vi "Delete TargetPanel by NodeRef.vi"(8 "error in":errorcluster caption="错误输入（无错误）", 9 "Abort VI":bool=TRUE, 10 "Node*":refnum<data-value>, 11 "PanelRootNode 输入":refnum<class "PanelRootNode.lvclass"> caption="DNL_LabVIEW Object in") -> (0 "error out":errorcluster caption="错误输出", 3 "PanelRootNode 输出":refnum<class "PanelRootNode.lvclass"> caption="DNL_LabVIEW Object out")   [LabVIEW 2013, in "PanelRootNode.lvclass"]
uses:
  PanelRootNode.lvclass
  PanelObject/PanelObject.lvclass
  PanelLinkNode/PanelLinkNode.lvclass/PanelLinkNode.ctl
  PanelDataNode/PanelDataNode.lvclass
  PanelLinkNode/PanelLinkNode.lvclass
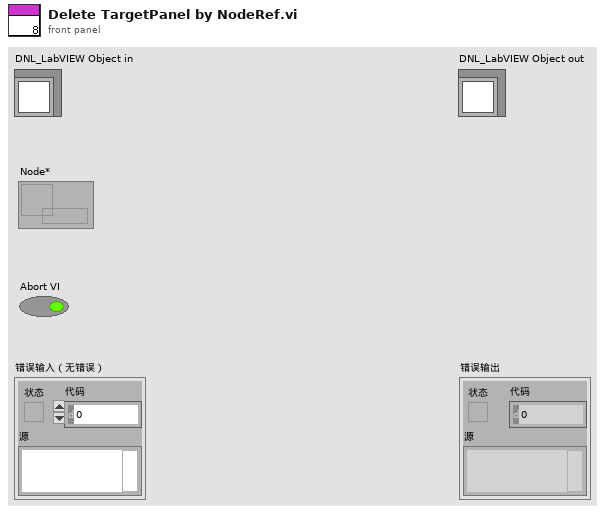
[diagram p1: front panel]
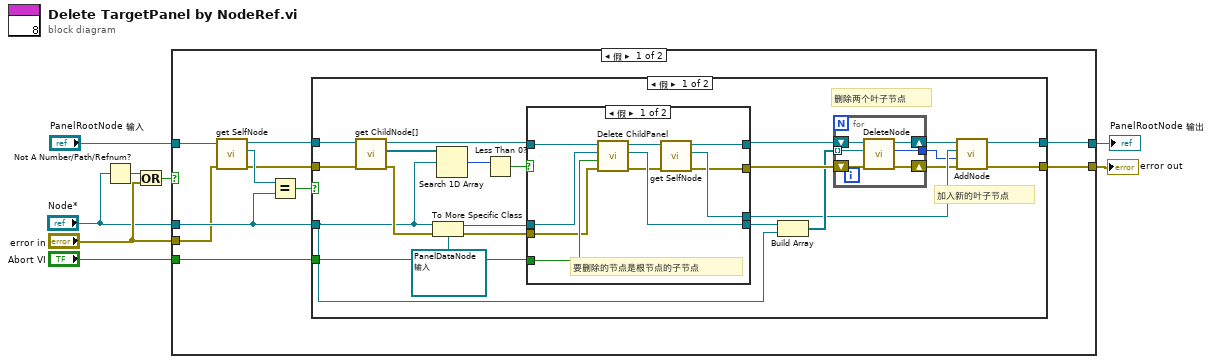
[diagram p0: block diagram]
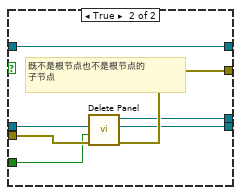
[diagram p2: hidden frame]
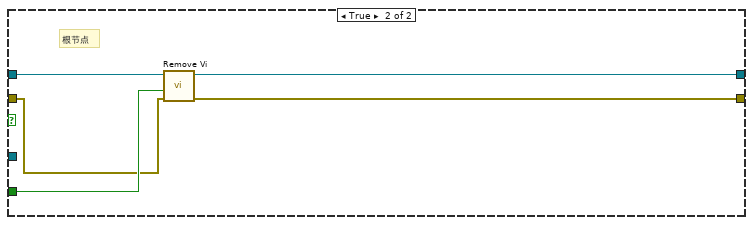
[diagram p3: hidden frame]
diagram:
  n1 = Not A Number/Path/Refnum?(number/path/refnum="Node*") -> (NaN/Path/Refnum?=w5:bool)
  n2 = Or(x=w5, y="error in") -> (x .or. y?=w4:bool)
  n3 = case shown="假" w4 {
    tunnel: [w10 w69] -> w8
    tunnel: [w14 w70] -> w6
    tunnel: "PanelRootNode 输入" -> [w18 w70]
    tunnel: "Node*" -> [w11 _]
    tunnel: "error in" -> [w9 w69]
    tunnel: "Abort VI" -> [w13 _]
    frame False {
      n4 = call "get SelfNode.vi"("error in (no error)"=w9, "PanelLinkNode输入"=w18) -> ("error out"=w12:errorcluster, "SelfNode*"=w17:refnum<data-value>, "PanelLinkNode输出"=w16:refnum<class "PanelRootNode.lvclass">)  [unwired: 7 in]
      n5 = Equal?(x=w17, y=w11) -> (x = y?=w15:bool)
      n6 = case shown="假" w15 {
        tunnel: w16 -> [w40 w68]
        tunnel: [w23 w67] -> w14
        tunnel: w13 -> [w34 w66]
        tunnel: w12 -> [w39 w64]
        tunnel: w11 -> [w27 _]
        tunnel: [w19 w65] -> w10
        frame False {
          # "加入新的叶子节点"
          # "删除两个叶子节点"
          n7 = call "get ChildNode[].vi"("error in (no error)"=w39, "PanelLinkNode输入"=w40) -> ("error out"=w31:errorcluster, "ChildNode*[]"=w38:refnum<data-value>[], "PanelLinkNode输出"=w36:refnum<class "PanelRootNode.lvclass">)  [unwired: 7 in]
          n8 = To More Specific Class(target class=refnum<data-value> refnum ("数据值引用"), reference=w27, error in=w31) -> (specific class reference=w32:refnum<data-value>, error out=w30:errorcluster)
          n9 = Search 1D Array(1D array=w38, element=w27) -> (index of element=w37:i32)  [unwired: 1 in]
          n10 = Less Than 0?(x=w37) -> (x < 0?=w35:bool)
          n11 = case shown="假" w35 {
            tunnel: w36 -> [w56 w63]
            tunnel: [w50 w63] -> w29
            tunnel: w32 -> [w55 w62]
            tunnel: w34 -> [w54 w59]
            tunnel: w30 -> [w53 w61]
            tunnel: [w47 w60] -> w26
            tunnel: [w52 w58] -> w28
            tunnel: [w49 w57] -> w22
            frame False {
              # "要删除的节点是根节点的子节点"
              n12 = call-dynamic "Delete ChildPanel.vi"("error in"=w53, "Abort VI"=w54, "ChildNode*"=w55, "ParentNode in"=w56) -> ("error out"=w48:errorcluster, "AnotherChildNode*"=w52:refnum<data-value>, "Parent out"=w51:refnum<class "PanelRootNode.lvclass">)  [unwired: 5 in]
              n13 = call "get SelfNode.vi"("error in (no error)"=w48, "PanelLinkNode输入"=w51) -> ("error out"=w47:errorcluster, "SelfNode*"=w49:refnum<data-value>, "PanelLinkNode输出"=w50:refnum<class "PanelRootNode.lvclass">)  [unwired: 7 in]
            }
            frame True {
              # "既不是根节点也不是根节点的\n子节点"
              n14 = call "Delete Panel.vi"("error in (no error)"=w61, "Abort VI"=w59, "SelfNode*"=w62) -> ("error out"=w60:errorcluster, "BrotherNodeBeDeleted"=w58:refnum<data-value>, "ParentNode*"=w57:refnum<data-value>)  [unwired: 6 in]
            }
          }
          n15 = Build Array(w28, w27) -> (w25:refnum<data-value>[])
          n16 = for {
            tunnel: w25 -> [w43] mode=indexing
            shift-right: [w45] -> w24
            shift-left: w29 -> [w46]
            shift-right: [w42] -> w20
            shift-left: w26 -> [w44]
            tunnel: [w41] -> w21
            n17 = call "DeleteNode.vi"("error in (no error)"=w44, "Node*"=w43, "PanelRootNode 输入"=w46) -> ("error out"=w42:errorcluster, "index"=w41:i32, "PanelRootNode 输出"=w45:refnum<class "PanelRootNode.lvclass">)  [unwired: 6 in]
          }
          n18 = call "AddNode.vi"("error in (no error)"=w20, "Index"=w21, "Node*"=w22, "PanelRootNode 输入"=w24) -> ("error out"=w19:errorcluster, "PanelRootNode 输出"=w23:refnum<class "PanelRootNode.lvclass">)  [unwired: 6 in]
        }
        frame True {
          # "根节点"
          n19 = call-dynamic "Remove Vi.vi"("error in"=w64, "Abort VI"=w66, "PanelDataNode 输入"=w68) -> ("error out"=w65:errorcluster, "PanelDataNode 输出"=w67:refnum<class "PanelRootNode.lvclass">)  [unwired: 5 in, 2 out]
        }
      }
    }
    frame True {
    }
  }
  "error out" <- w8
  "PanelRootNode 输出" <- w6
